vi "Setup Maps and Queues.vi"(8 "error in (no error)":errorcluster, 11 "WAMP Client in":refnum<class "WAMP Client.lvclass">) -> (0 "error out":errorcluster, 3 "WAMP Client out":refnum<class "WAMP Client.lvclass">)   [LabVIEW 2020, in "wamplv.lvlib" / "WAMP Client.lvclass"]
uses:
  WAMP Client.lvclass
  TypeDef/Write queue item.ctl
  TypeDef/EVENT payload.ctl
  API/TypeDefs/RESULT payload (JSON).ctl
  API/TypeDefs/Combined error.ctl
  API/TypeDefs/WAMP error.ctl
  API/TypeDefs/INVOCATION payload.ctl
  Private/Invocation Request ID/Invocation Request ID.lvclass
  TypeDef/Internal Message.ctl
  TypeDef/Internal Message Type.ctl
  TypeDef/Termination Request.ctl
  API/TypeDefs/Termination Reason.ctl
  TypeDef/Termination Reason Enum.ctl
  API/TypeDefs/Disconnected event data.ctl
  API/TypeDefs/Connected event data.ctl
  TypeDef/Message Loop Data.ctl
  TypeDef/REGISTER Request Data.ctl
  TypeDef/Success or error.ctl
  TypeDef/Publish Requests Map.ctl
  TypeDef/PUBLISH Request Data.ctl
  TypeDef/PUBLISH result.ctl
  TypeDef/Endpoint Data.ctl
  TypeDef/CALL Request Map.ctl
  Private/Requests/ICallRequest/ICallRequest.lvclass
  TypeDef/SUBSCRIBE Requests Map.ctl
  TypeDef/SUBSCRIBE Request Data.ctl
  TypeDef/Subscribe Result.ctl
  TypeDef/Subscriptions Map.ctl
  TypeDef/Subscription Details.ctl
  TypeDef/Unsubscribe Requests Map.ctl
  TypeDef/UNSUBSCRIBE Request Data.ctl
  TypeDef/UNSUBSCRIBE Result.ctl
  TypeDef/Unregister requests map.ctl
  TypeDef/Unregister request.ctl
  WAMP Client.lvclass/WAMP Client.ctl
  <vilib>/ErrorRing/Error Ring.xnode
  wamplv.lvlib
  Private/TypeDefs/Transport type.ctl
panel:
  in  "queue out":refnum<queue>
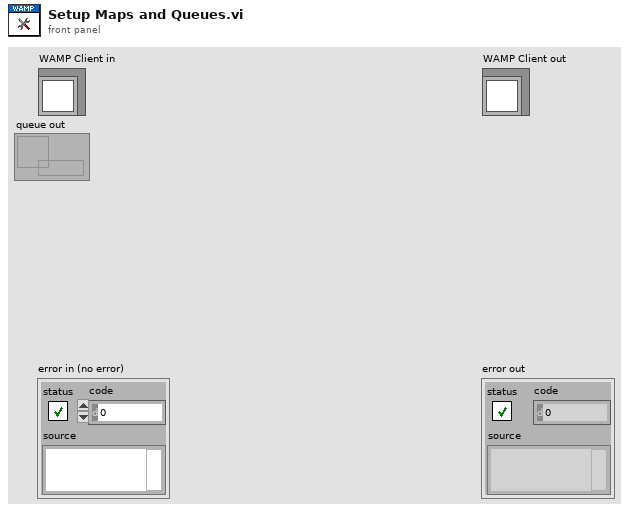
[diagram p1: front panel]
types:
  T1 = typedef "wamplv.lvlib/Write queue item.ctl" = cluster{"Type":T2, "String":string, "Bytes":u8[]}
  T2 = typedef "wamplv.lvlib/Transport type.ctl" = enum16{"Binary", "Text"}
  T3 = typedef "wamplv.lvlib/WAMP Client.lvclass/Message Loop Data.ctl" = cluster{"Last Request ID":u64, "Register Requests":map{u64, T4}, "Publish Requests":T5, "Endpoints Map":map{u64, T7}, "Call Requests":T8, "Subscription Requests":T9, "Subscriptions":T11, "Unsubscribe Requests":T13, "Random Request IDs":u64[], "Unregister requests map":T15}
  T4 = typedef "wamplv.lvlib/WAMP Client.lvclass/REGISTER Request Data.ctl" = cluster{"Procedure URI":string, "Options":string, "REGISTER result notifier":refnum<notifier>}
  T5 = typedef "wamplv.lvlib/WAMP Client.lvclass/Publish Requests Map.ctl" = map{u64, T6}
  T6 = typedef "wamplv.lvlib/WAMP Client.lvclass/PUBLISH Request Data.ctl" = cluster{"Topic URI":string, "Arguments":string, "ArgumentsKw":string, "Request Acknowledgement":bool, "Options":string, "Publish result notifier":refnum<notifier>}
  T7 = typedef "wamplv.lvlib/WAMP Client.lvclass/Endpoint Data.ctl" = cluster{"Procedure URI":string}
  T8 = typedef "wamplv.lvlib/WAMP Client.lvclass/CALL Request Map.ctl" = map{u64, refnum<class "ICallRequest.lvclass">}
  T9 = typedef "wamplv.lvlib/WAMP Client.lvclass/SUBSCRIBE Requests Map.ctl" = map{u64, T10}
  T10 = typedef "wamplv.lvlib/WAMP Client.lvclass/SUBSCRIBE Request Data.ctl" = cluster{"Topic":string, "Subscribe result notifer":refnum<notifier>, "Options":string}
  T11 = typedef "wamplv.lvlib/WAMP Client.lvclass/Subscriptions Map.ctl" = map{u64, T12}
  T12 = typedef "wamplv.lvlib/WAMP Client.lvclass/Subscription Details.ctl" = cluster{"Subscription ID":u64, "Topic":string, "Publication Received Event":refnum<user-event>, "Publication Received Notifier":refnum<notifier>, "Number of subscriptions":u64}
  T13 = typedef "wamplv.lvlib/WAMP Client.lvclass/Unsubscribe Requests Map.ctl" = map{u64, T14}
  T14 = typedef "wamplv.lvlib/WAMP Client.lvclass/UNSUBSCRIBE Request Data.ctl" = cluster{"Topic":string, "Unsubscrube result notifier":refnum<notifier>, "Options":string}
  T15 = typedef "wamplv.lvlib/WAMP Client.lvclass/Unregister requests map.ctl" = map{u64, T16}
  T16 = typedef "wamplv.lvlib/WAMP Client.lvclass/Unregister request.ctl" = cluster{"URI":string, "Unregister result notifier":refnum<notifier>, "Options":string}
  T17 = typedef "wamplv.lvlib/WAMP Client.lvclass/Connected event data.ctl" = cluster{"Session ID":u64}
  T18 = typedef "wamplv.lvlib/WAMP Client.lvclass/Disconnected event data.ctl" = cluster{"Termination Reason":T19, "Error Out":errorcluster}
  T19 = typedef "wamplv.lvlib/WAMP Client.lvclass/Termination Reason.ctl" = cluster{"Reason":T20, "Reason URI":string, "Message":string}
  T20 = typedef "wamplv.lvlib/WAMP Client.lvclass/Termination Reason Enum.ctl" = enum16{"Goodbye Received", "Abort Received", "Send Goodbye", "Send Abort", "Read Loop Failure", "Write Loop Failure", "Message Loop Failure", "wamplv aborted"}
  T21 = typedef "wamplv.lvlib/WAMP Client.lvclass/Termination Request.ctl" = cluster{"Terminate?":bool, "Termination Reason":T19}
  T22 = typedef "wamplv.lvlib/WAMP Client.lvclass/Internal Message.ctl" = cluster{"Internal Message Type":T23, "Variant":variant}
  T23 = typedef "wamplv.lvlib/WAMP Client.lvclass/Internal Message Type.ctl" = enum16{"Subscribe", "Handle Subscribed", "Handle Event", "Unsubscribe", "Handle Unsubscribed", "Publish", "Handled Published", "Goodbye", "Handle Goodbye", "Call", "Handle Result", "Register", "Handle Registered", "Unregister", "Handle Unregistered", "Handle Invocation", "Yield", "Error"}
  T24 = typedef "wamplv.lvlib/WAMP Client.lvclass/EVENT payload.ctl" = cluster{"Arguments Payload":string, "ArgumentKw Payload":string, "Topic":string}
  T25 = typedef "wamplv.lvlib/WAMP Client.lvclass/INVOCATION payload.ctl" = cluster{"Arguments":string, "ArgumentKw":string, "Procedure URI":string, "Details":string, "Registration ID":u64, "Invocation Request ID":refnum<class "Invocation Request ID.lvclass">}
  T26 = typedef "wamplv.lvlib/WAMP Client.lvclass/RESULT payload (JSON).ctl" = cluster{"Arguments Payload":string, "ArgumentKw Payload":string, "Topic":string, "Combined Error":T27}
  T27 = typedef "wamplv.lvlib/WAMP Client.lvclass/Combined error.ctl" = cluster{"Error?":bool, "WAMP Error":T28, "Error":errorcluster}
  T28 = typedef "wamplv.lvlib/WAMP Client.lvclass/WAMP error.ctl" = cluster{"Details":string, "ArgumentKw Payload":string, "Error?":bool, "Error URI":string, "Arguments Payload":string}
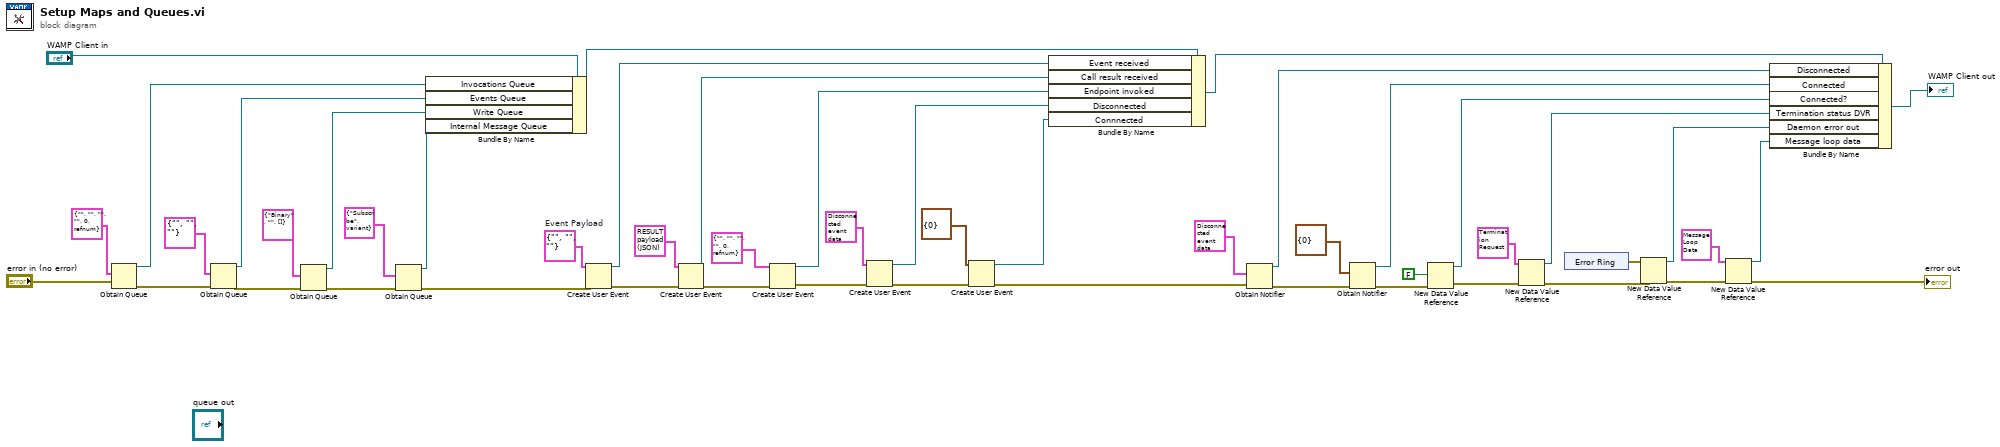
[diagram p0: block diagram]
diagram:
  w50 = T24 {"Arguments Payload"="", "ArgumentKw Payload"="", "Topic"=""}  # Event Payload
  n1 = Obtain Queue(element data type=T25 {"Arguments"="", "ArgumentKw"="", "Procedure URI"="", "Details"="", "Registration ID"=0, "Invocation Request ID"=refnum} ("INVOCATION payload"), error in (no error)="error in (no error)") -> (queue out=w33:refnum<queue>, error out=w41:errorcluster)  [unwired: 3 in, 1 out]
  n2 = Obtain Queue(element data type=T24 {"Arguments Payload"="", "ArgumentKw Payload"="", "Topic"=""} ("Cluster"), error in (no error)=w41) -> (queue out=w32:refnum<queue>, error out=w24:errorcluster)  [unwired: 3 in, 1 out]
  n3 = Obtain Queue(element data type=T1 {"Type"=enum."Binary", "String"="", "Bytes"=[]} ("Cluster"), error in (no error)=w24) -> (queue out=w2:refnum<queue>, error out=w25:errorcluster)  [unwired: 3 in, 1 out]
  n4 = Obtain Queue(element data type=T22 {"Internal Message Type"=enum."Subscribe", "Variant"=variant} ("Cluster"), error in (no error)=w25) -> (queue out=w26:refnum<queue>, error out=w11:errorcluster)  [unwired: 3 in, 1 out]
  n5 = Bundle By Name(cluster="WAMP Client in", "Invocations Queue"=w33, "Events Queue"=w32, "Write Queue"=w2, "Internal Message Queue"=w26) -> (w30:refnum<class "WAMP Client.lvclass">)
  n6 = Create User Event(user event datatype=w50, error in=w11) -> (user event=w29:refnum<user-event>, error out=w47:errorcluster)
  n7 = Create User Event(user event datatype=T26 {"Arguments Payload"="", "ArgumentKw Payload"="", "Topic"="", "Combined Error"={"Error?"=FALSE, "WAMP Error"={"Details"="{}", "ArgumentKw Payload"="", "Error?"=FALSE, "Error URI"="", "Arguments Payload"=""}, "Error"={"status"=FALSE, "code"=0, "source"=""}}} ("RESULT Payload"), error in=w47) -> (user event=w28:refnum<user-event>, error out=w44:errorcluster)
  n8 = Create User Event(user event datatype=T25 {"Arguments"="", "ArgumentKw"="", "Procedure URI"="", "Details"="", "Registration ID"=0, "Invocation Request ID"=refnum} ("INVOCATION payload"), error in=w44) -> (user event=w27:refnum<user-event>, error out=w17:errorcluster)
  n9 = Create User Event(user event datatype=T18 {"Termination Reason"={"Reason"=enum."Goodbye Received", "Reason URI"="wamp.error.protocol_violation", "Message"=""}, "Error Out"={"status"=FALSE, "code"=0, "source"=""}} ("Cluster"), error in=w17) -> (user event=w14:refnum<user-event>, error out=w15:errorcluster)
  n10 = Create User Event(user event datatype=T17 {"Session ID"=0} ("Connected event data"), error in=w15) -> (user event=w13:refnum<user-event>, error out=w12:errorcluster)
  n11 = Bundle By Name(cluster=w30, "Event received"=w29, "Call result received"=w28, "Endpoint invoked"=w27, "Disconnected"=w14, "Connnected"=w13) -> (w23:refnum<class "WAMP Client.lvclass">)
  n12 = Obtain Notifier(notification data type=T18 {"Termination Reason"={"Reason"=enum."Goodbye Received", "Reason URI"="wamp.error.protocol_violation", "Message"=""}, "Error Out"={"status"=FALSE, "code"=0, "source"=""}} ("Cluster"), error in (no error)=w12) -> (notifier out=w34:refnum<notifier>, error out=w21:errorcluster)  [unwired: 2 in, 1 out]
  n13 = Obtain Notifier(notification data type=T17 {"Session ID"=0} ("Connected event data"), error in (no error)=w21) -> (notifier out=w19:refnum<notifier>, error out=w22:errorcluster)  [unwired: 2 in, 1 out]
  n14 = New Data Value Reference(data value=FALSE, error in=w22) -> (data value reference=w38:refnum<data-value>, error out=w36:errorcluster)
  n15 = New Data Value Reference(data value=T21 {"Terminate?"=FALSE, "Termination Reason"={"Reason"=enum."Goodbye Received", "Reason URI"="wamp.error.protocol_violation", "Message"=""}} ("Daemon Termination Request"), error in=w36) -> (data value reference=w37:refnum<data-value>, error out=w10:errorcluster)
  n16 = xnode "Error Ring"() -> ("error out"=w9:errorcluster)
  n17 = New Data Value Reference(data value=w9, error in=w10) -> (data value reference=w8:refnum<data-value>, error out=w6:errorcluster)
  n18 = New Data Value Reference(data value=T3 {"Last Request ID"=0, "Register Requests"={}, "Publish Requests"={}, "Endpoints Map"={}, "Call Requests"={}, "Subscription Requests"={}, "Subscriptions"={}, "Unsubscribe Requests"={}, "Random Request IDs"=[], "Unregister requests map"={}} ("Message Loop Shift Register Data"), error in=w6) -> (data value reference=w5:refnum<data-value>, error out=→"error out":errorcluster)
  n19 = Bundle By Name(cluster=w23, "Disconnected"=w34, "Connected"=w19, "Connected?"=w38, "Termination status DVR"=w37, "Daemon error out"=w8, "Message loop data"=w5) -> (→"WAMP Client out":refnum<class "WAMP Client.lvclass">)
